vi "Find Homography.vi"(7 "USAC Params (Default: OpenCV Defaults) in":refnum<class "USAC Params.lvclass">, 8 "error in (no error)":errorcluster, 10 "Target Points":T2[](array[typedef]), 11 "Source Points":T2[](array[typedef])) -> (0 "error out":errorcluster, 3 "Homography Matrix":T1, 4 "Inliers":i32[](array[numeric]))   [LabVIEW 2020, in "ar.lvlib"]
doc: "Compute the homography that maps between matching 2D pointsets between two planes. \n\nThe function is tolerant of noisy and incorrect point correspondence via use of USAC outlier rejection and optimization. See https://docs.opencv.org/4.10.0/de/d3e/tutorial_usac.html for more information on the USAC parameters."
uses:
  ar.lvlib
  common/Image Point (Float).ctl
  USAC Params/USAC Params.lvclass
  <vilib>/Analysis/Matrix/Datatypes/RealMatrix.ctl
  USAC Params/USAC Params.lvclass/USAC Params.ctl
  common/Object Point (Float).ctl
  <vilib>/Analysis/Matrix/Numeric/Conversions/Array To Matrix - RA2.vi
  common/common.lvlib
  <vilib>/Analysis/Matrix/NI_Matrix.lvlib
  common/bin/gartoolkit_ar_32-1.dll
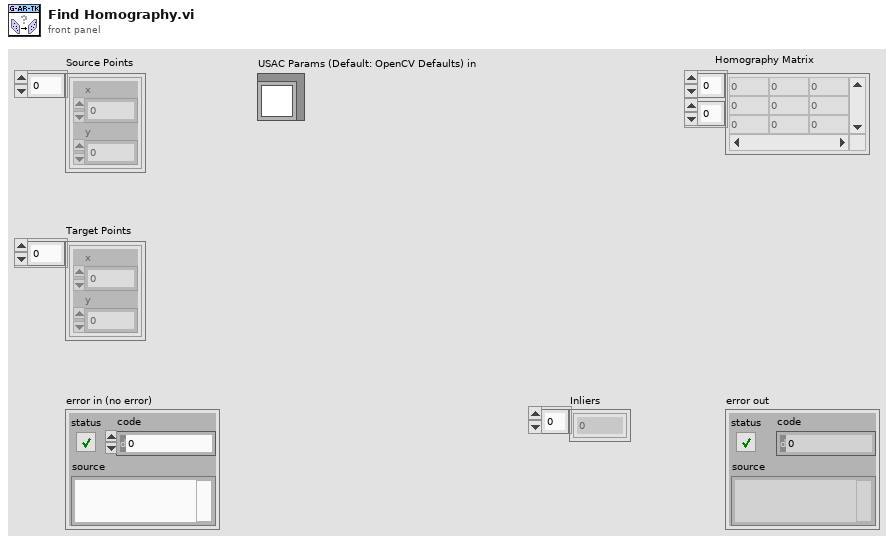
[diagram p1: front panel]
types:
  T1 = typedef "NI_Matrix.lvlib/RealMatrix.ctl" = dbl[][]
  T2 = typedef "common.lvlib/Image Point (Float).ctl" = cluster{"x":dbl, "y":dbl}
  T3 = typedef "common.lvlib/Object Point (Float).ctl" = cluster{"x":dbl, "y":dbl, "z":dbl}
  T4 = typedef "ar.lvlib/USAC Params.lvclass/Parameters.ctl" = cluster{"Confidence":dbl, "Threshold":dbl, "Final Polisher Iterations":u16, "Local Optimization Iterations":u16, "Local Optimization Sample Size":u16, "Max Iterations":u16, "Random Generator State":i32, "Final Polisher":T5, "Local Optimization Method":T6, "Neighbor Search Method":T7, "Sampler":T8, "Score":T9, "Is Parallel":bool}
  T5 = typedef "ar.lvlib/USAC Params.lvclass/Polishing Methods.ctl" = enum8{"NONE", "LSQ", "MAGSAC", "COV"}
  T6 = typedef "ar.lvlib/USAC Params.lvclass/Local Optimization Methods.ctl" = enum8{"NULL", "INNER_LO", "INNER_AND_ITER_LO", "GC", "SIGMA"}
  T7 = typedef "ar.lvlib/USAC Params.lvclass/Neighbor Search Methods.ctl" = enum8{"FLANN_KNN", "GRID", "FLANN_RADIUS"}
  T8 = typedef "ar.lvlib/USAC Params.lvclass/Sampling Methods.ctl" = enum8{"UNIFORM", "PROGRESSIVE_NAPSAC", "NAPSAC", "PROSAC"}
  T9 = typedef "ar.lvlib/USAC Params.lvclass/Score Methods.ctl" = enum8{"RANSAC", "MSAC", "MAGSAC", "LMEDS"}
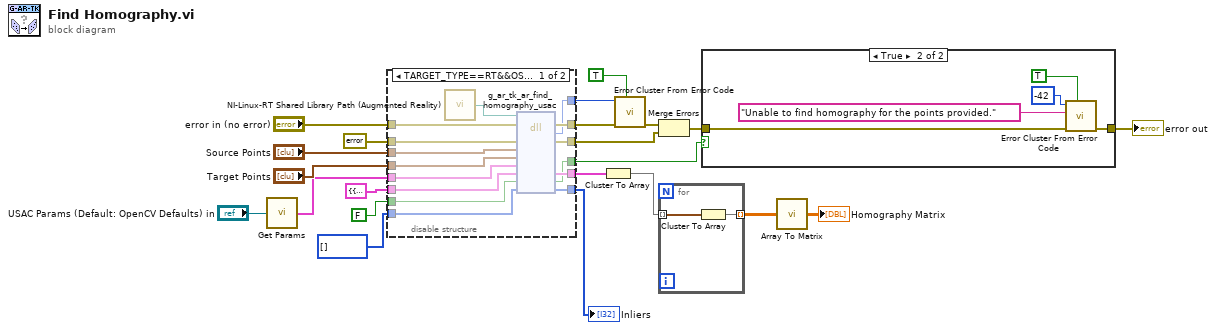
[diagram p0: block diagram]
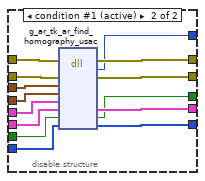
[diagram p3: hidden frame]
diagram:
  n1 = call "Get Params.vi"("USAC Params in"="USAC Params (Default: OpenCV Defaults) in") -> ("Parameters"=w13:T4)
  n2 = disable-structure shown="TARGET_TYPE==RT&&OS==Linux" {
    disable-tunnel: "error in (no error)" -> [w36 w51]
    disable-tunnel: errorcluster {"status"=FALSE, "code"=0, "source"=""} ("error constant") -> [w35 w47]
    disable-tunnel: [w28 w50] -> w21
    disable-tunnel: [w27 w49] -> w19
    disable-tunnel: [w26 w48] -> w20
    disable-tunnel: "Source Points" -> [w34 w46]
    disable-tunnel: "Target Points" -> [w33 w45]
    disable-tunnel: w13 -> [w32 w44]
    disable-tunnel: cluster{"[0]":T3, "[1]":T3, "[3]":T3} {"[0]"={"x"=0.0, "y"=0.0, "z"=0.0}, "[1]"={"x"=0.0, "y"=0.0, "z"=0.0}, "[3]"={"x"=0.0, "y"=0.0, "z"=0.0}} -> [w31 w43]
    disable-tunnel: [w25 w42] -> w11
    disable-tunnel: FALSE -> [w30 w41]
    disable-tunnel: i32[] [] ("inliers") -> [w29 w40]
    disable-tunnel: [w24 w39] -> w5
    disable-tunnel: [w23 w38] -> w2
    frame condition #0 {
      n3 = call "NI-Linux-RT Shared Library Path (Augmented Reality).vi"() -> ("Path"=w37:path)
      n4 = dll-call lib="?" fn="g_ar_tk_ar_find_homography_usac" ("g_ar_toolkit.*.*:g_ar_tk_image_copy")(path in=w37, error in=w36, "error_cluster"=w35, "source_points"=w34, "target_points"=w33, "usac_params"=w32, "h"=w31, "is_empty"=w30, "inliers"=w29) -> (error out=w28:errorcluster, w27:i32, "error_cluster"=w26:errorcluster, "h"=w25:cluster{"[0]":T3, "[1]":T3, "[3]":T3}, "is_empty"=w23:bool, "inliers"=w24:i32[])  [unwired: 4 in, 1 out]
    }
    frame condition #1 (active) {
      n5 = dll-call lib="C:/serenial/lib/g-augmented-reality-toolkit/LabVIEW/common/bin/gartoolkit_ar_*-1.*" fn="g_ar_tk_ar_find_homography_usac" ("g_ar_toolkit.*.*:g_ar_tk_image_copy")(error in=w51, "error_cluster"=w47, "source_points"=w46, "target_points"=w45, "usac_params"=w44, "h"=w43, "is_empty"=w41, "inliers"=w40) -> (error out=w50:errorcluster, w49:i32, "error_cluster"=w48:errorcluster, "h"=w42:cluster{"[0]":T3, "[1]":T3, "[3]":T3}, "is_empty"=w38:bool, "inliers"=w39:i32[])  [unwired: 5 in, 1 out]
    }
  }
  "Inliers" <- w5
  n6 = Cluster To Array(cluster=w11) -> (array=w10:T3[])
  n7 = call <vilib>:"Error Cluster From Error Code.vi"("show call chain? (False)"=TRUE, "error in (no error)"=w21, "error code (0)"=w19) -> ("error out"=w22:errorcluster)  [unwired: 6 in]
  n8 = Merge Errors(w22, w20) -> (w3:errorcluster)
  n9 = for {
    tunnel: w10 -> [w53] mode=indexing
    tunnel: [w52] -> w9 mode=indexing
    n10 = Cluster To Array(cluster=w53) -> (array=w52:dbl[])
  }
  n11 = case shown="True" w2 {
    tunnel: [w54 w58] -> w4
    tunnel: w3 -> [w54 w59]
    frame False {
    }
    frame True {
      n12 = call <vilib>:"Error Cluster From Error Code.vi"("show call chain? (False)"=TRUE, "error in (no error)"=w59, "error message (\"\")"="Unable to find homography for the points provided." ("error message (\"\")"), "error code (0)"=-42) -> ("error out"=w58:errorcluster)  [unwired: 5 in]
    }
  }
  "error out" <- w4
  n13 = call-poly <vilib>:"Array To Matrix.vi"("Real 2D Array"=w9) -> ("Real Matrix"=→"Homography Matrix":T1)
